vi "CurveDisplay.vi"(8 "曲线点数":i32=10 caption="显示时长" min=1 step=1, 9 "时间单位":enum16{"秒", "分钟", "小时"}(ring), 10 "时间显示":bool, 11 "数据":T1) -> (2 "图形输出":cluster{"数组":dbl[], "数组":dbl[]}[](array[cluster]), 3 "数据输出":cluster{"数组":dbl[]}[](array[cluster]))   [LabVIEW 2018, in "DataDisplay.lvlib" / "TrendPlot.lvclass"]
uses:
  TrendPlot.lvclass
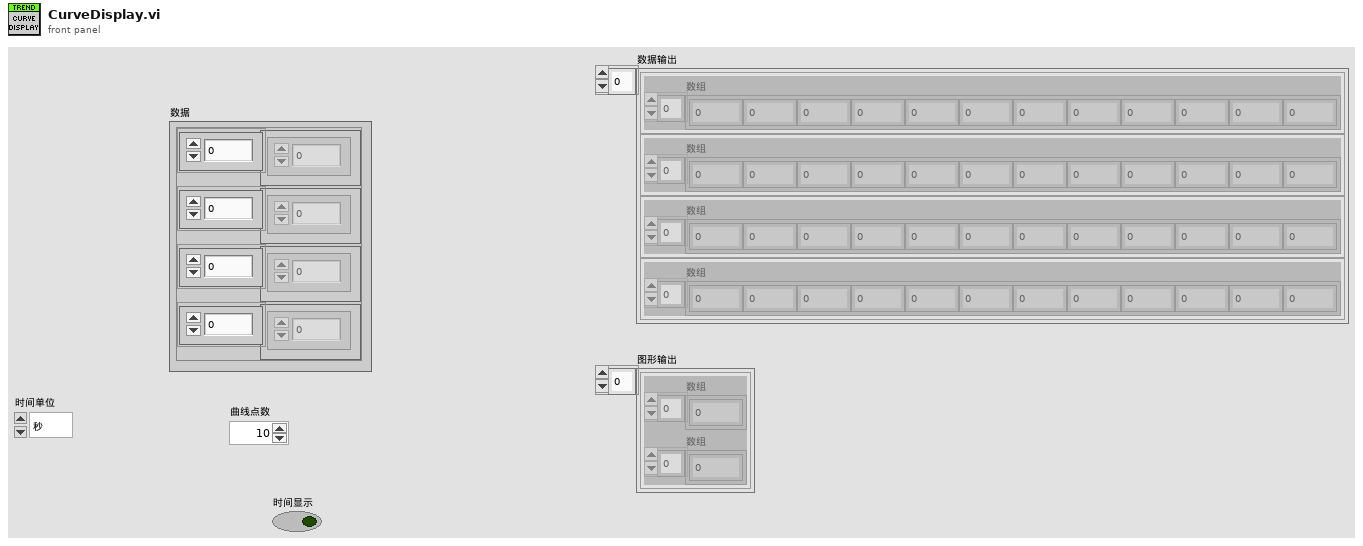
[diagram p1: front panel]
types:
  T1 = cluster{"数组":dbl[], "数组":dbl[], "数组":dbl[], "数组":dbl[]}
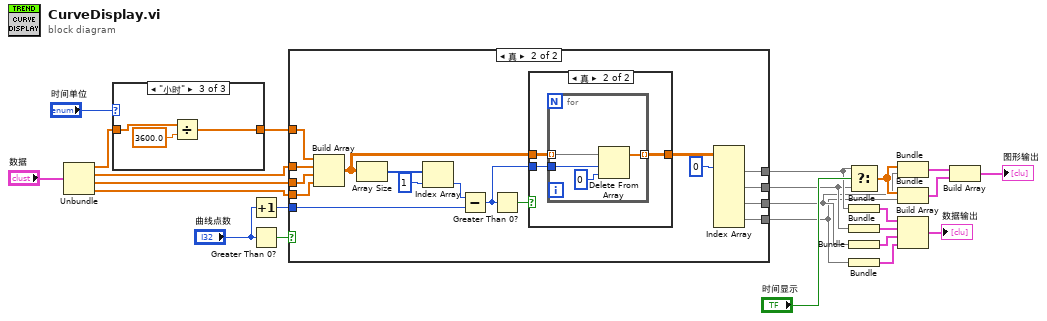
[diagram p0: block diagram]
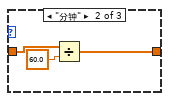
[diagram p5: hidden frame]
diagram:
  n1 = Unbundle("数据") -> ("数组"=w21:dbl[], "数组"=w11:dbl[], "数组"=w17:dbl[], "数组"=w16:dbl[])
  n2 = case shown="\"小时\"" "时间单位" {
    tunnel: [w25 w28 w31] -> w12
    tunnel: w21 -> [w25 w27 w30]
    frame "秒", Default {
    }
    frame "分钟" {
      n3 = Divide(x=w27, y=60.0) -> (x/y=w28:dbl[])
    }
    frame "小时" {
      n4 = Divide(x=w30, y=3600.0) -> (x/y=w31:dbl[])
    }
  }
  n5 = Increment(x="曲线点数") -> (x+1=w13:i32)
  n6 = Greater Than 0?(x="曲线点数") -> (x > 0?=w14:bool)
  n7 = case shown="真" w14 {
    tunnel: w11 -> [w35 w52]
    tunnel: w17 -> [w34 w51]
    tunnel: w16 -> [w33 w50]
    tunnel: w13 -> [_ w46]
    tunnel: [w35 w41] -> w8
    tunnel: [w34 w40] -> w5
    tunnel: [w33 w39] -> w4
    tunnel: w12 -> [w32 w38]
    tunnel: [w32 w36] -> w9
    frame False {
    }
    frame True {
      n8 = Build Array(w38, w52, w51, w50) -> (w44:dbl[][])
      n9 = Array Size(array=w44) -> (size(s)=w49:i32[])
      n10 = Index Array(array=w49, index=1 ("索引")) -> (element=w47:i32)
      n11 = Subtract(x=w47, y=w46) -> (x-y=w43:i32)
      n12 = Greater Than 0?(x=w43) -> (x > 0?=w45:bool)
      n13 = case shown="真" w45 {
        tunnel: w44 -> [w53 w56]
        tunnel: w43 -> [_ w55]
        tunnel: [w53 w54] -> w42
        frame False {
        }
        frame True {
          n14 = for {
            tunnel: w56 -> [w60] mode=indexing
            tunnel: w55 -> [w59]
            tunnel: [w57] -> w54 mode=indexing
            n15 = Delete From Array(array=w60, length=w59, index=0 ("索引")) -> (array with subset deleted=w57:dbl[])  [unwired: 1 out]
          }
        }
      }
      n16 = Index Array(array=w42, index (row) #1=0 ("索引 (行)")) -> (element #1=w36:dbl[], element #2=w41:dbl[], element #3=w40:dbl[], element #4=w39:dbl[])  [unwired: 7 in]
    }
  }
  n17 = Select(t=w9, s="时间显示", f=w8) -> (s? t:f=w10:dbl[])
  n18 = Bundle("数组"=w9) -> (w7:cluster{"数组":dbl[]})  [unwired: 1 in]
  n19 = Bundle("数组"=w8) -> (w6:cluster{"数组":dbl[]})  [unwired: 1 in]
  n20 = Bundle("数组"=w5) -> (w3:cluster{"数组":dbl[]})  [unwired: 1 in]
  n21 = Bundle("数组"=w4) -> (w2:cluster{"数组":dbl[]})  [unwired: 1 in]
  n22 = Bundle("数组"=w10, "数组"=w5) -> (w24:cluster{"数组":dbl[], "数组":dbl[]})  [unwired: 1 in]
  n23 = Bundle("数组"=w10, "数组"=w4) -> (w23:cluster{"数组":dbl[], "数组":dbl[]})  [unwired: 1 in]
  n24 = Build Array(w7, w6, w3, w2) -> (→"数据输出":cluster{"数组":dbl[]}[])
  n25 = Build Array(w24, w23) -> (→"图形输出":cluster{"数组":dbl[], "数组":dbl[]}[])
